vi "AllowEdgeStartCheck.vi"(0 "reference in":refnum<class "StateDiagramGraph.lvclass">, 1 "EdgeStartNode":refnum<class "AbstractNode.lvclass">, 2 "GraphButton":u32, 5 "error in (no error)":errorcluster) -> (14 "reference out":refnum<class "StateDiagramGraph.lvclass">, 16 "Allowed":bool, 19 "error out":errorcluster)   [LabVIEW 2016, in "StateDiagramGraph.lvclass"]
uses:
  <resource>/Framework/Providers/Open_GDS/UML/StateDiagramGraph_class/StateDiagramGraph.lvclass
  <resource>/Framework/Providers/Open_GDS/UML/AbstractNode_class/AbstractNode.lvclass
  <resource>/Framework/Providers/Open_GDS/UML/AbstractEdge_class/AbstractEdge.lvclass
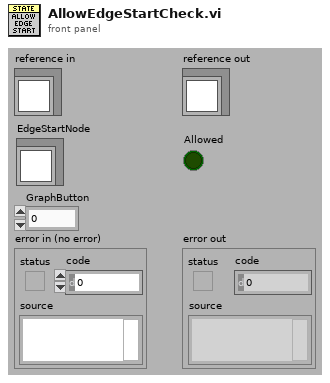
[diagram p1: front panel]
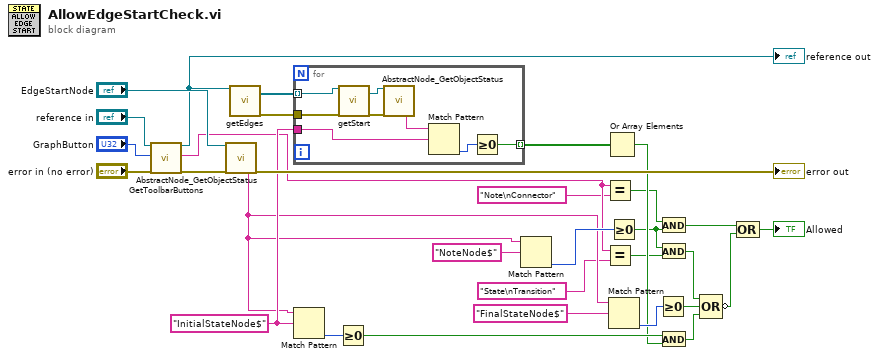
[diagram p0: block diagram]
diagram:
  w21 = "InitialStateNode$" ("regular expression")
  n1 = call-dynamic "GetToolbarButtons.vi"("reference in"="reference in", "GraphButton"="GraphButton", "error in (no error)"="error in (no error)") -> ("reference out"=w4:refnum<class "StateDiagramGraph.lvclass">, "Text"=w3:string, "error out"=w26:errorcluster)  [unwired: 12 in, 2 out]
  "reference out" <- w4
  n2 = call <resource>:"AbstractNode_GetObjectStatus.vi"("reference in"="EdgeStartNode", "error in (no error)"=w26) -> ("Class name"=w5:string, "error out"=→"error out":errorcluster)  [unwired: 16 out]
  n3 = call-dynamic "getEdges.vi"("reference"=w4) -> ("edges"=w19:refnum<class "AbstractEdge.lvclass">[], "error out"=w20:errorcluster)  [unwired: 16 in, 1 out]
  n4 = for {
    tunnel: w20 -> [w39]
    tunnel: w21 -> [w38]
    tunnel: [w36] -> w18 mode=indexing
    tunnel: w19 -> [w35] mode=indexing
    n5 = call-dynamic "getStart.vi"("reference"=w35, "error in (no error)"=w39) -> ("startNode"=w34:refnum<class "AbstractNode.lvclass">, "error out"=w33:errorcluster)  [unwired: 14 in, 2 out]
    n6 = call <resource>:"AbstractNode_GetObjectStatus.vi"("reference in"=w34, "error in (no error)"=w33) -> ("Class name"=w32:string)  [unwired: 17 out]
    n7 = Match Pattern(string=w32, regular expression=w38) -> (offset past match=w37:i32)  [unwired: 4 out]
    n8 = Greater Or Equal To 0?(x=w37) -> (x >= 0?=w36:bool)
  }
  n9 = Match Pattern(string=w5, regular expression=w21) -> (offset past match=w23:i32)  [unwired: 4 out]
  n10 = Greater Or Equal To 0?(x=w23) -> (x >= 0?=w17:bool)
  n11 = Match Pattern(string=w5, regular expression="NoteNode$") -> (offset past match=w12:i32)  [unwired: 4 out]
  n12 = Equal?(x=w3, y="Note\nConnector" ("Text")) -> (x = y?=w11:bool)
  n13 = Equal?(x=w3, y="State\nTransition" ("Text")) -> (x = y?=w8:bool)
  n14 = Or Array Elements(Boolean array=w18) -> (logical OR=w16:bool)
  n15 = Greater Or Equal To 0?(x=w12) -> (x >= 0?=w9:bool)
  n16 = Match Pattern(string=w5, regular expression="FinalStateNode$") -> (offset past match=w24:i32)  [unwired: 4 out]
  n17 = Greater Or Equal To 0?(x=w24) -> (x >= 0?=w22:bool)
  n18 = And(x=w11, y=w9) -> (x .and. y?=w10:bool)
  n19 = And(x=w9, y=w8) -> (x .and. y?=w7:bool)
  n20 = And(x=w17, y=w16) -> (x .and. y?=w15:bool)
  n21 = Compound Arithmetic op=OR(w7, w22, w15) -> (invert w14:bool)
  n22 = Compound Arithmetic op=OR(w10, w14) -> (→"Allowed":bool)
